vi "Read Type.vi"(8 "error in (no error)":errorcluster, 11 "MovementInstruction in":refnum<class "MovementInstruction.lvclass">) -> (0 "error out":errorcluster, 2 "Type":string, 3 "MovementInstruction out":refnum<class "MovementInstruction.lvclass">)   [LabVIEW 2015, in "MovementInstruction.lvclass"]
uses:
  MovementInstruction.lvclass
  Instruction.lvclass
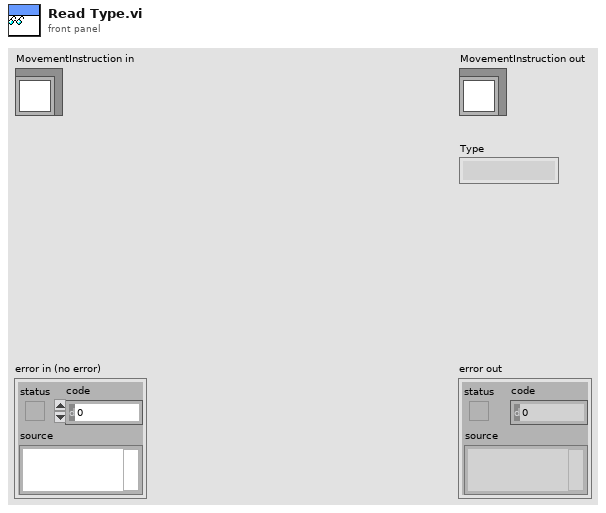
[diagram p1: front panel]
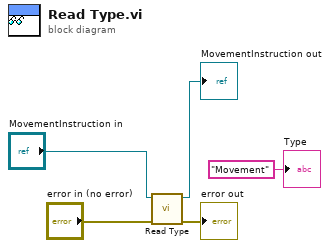
[diagram p0: block diagram]
diagram:
  n1 = call-parent "Read Type.vi"("error in (no error)"="error in (no error)", "Instruction in"="MovementInstruction in") -> ("error out"=→"error out":errorcluster, "Instruction out"=→"MovementInstruction out":refnum<class "MovementInstruction.lvclass">)  [unwired: 7 in, 1 out]
  "Type" <- "Movement" ("Type")
